vi "9604 String to Integer Overflow--error.vi"(7 "Type":T1(ring), 8 "error in":errorcluster, 11 "Integer String":string) -> (0 "error out":errorcluster)   [LabVIEW 2020, in "CANopen.lvlib"]
uses:
  CANopen.lvlib
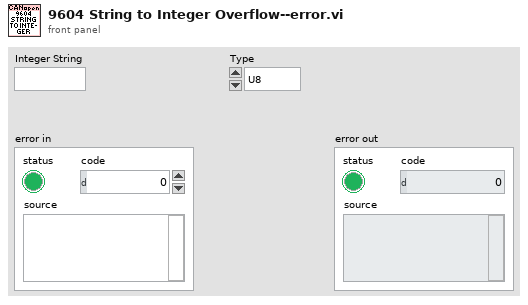
[diagram p1: front panel]
types:
  T1 = enum16{"U8", "U16", "U32", "I8", "I16", "I32", "I64", "U64"}
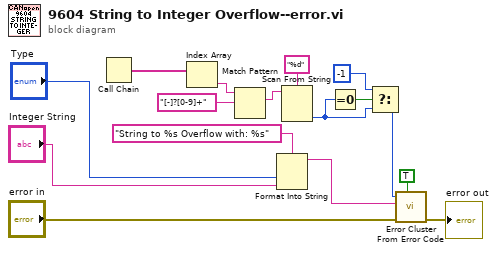
[diagram p0: block diagram]
diagram:
  n1 = Call Chain() -> (call chain=w9:string[])
  n2 = Index Array(array=w9) -> (element=w3:string)  [unwired: 1 in]
  n3 = Match Pattern(string=w3, regular expression="[-]?[0-9]+") -> (match substring=w2:string)  [unwired: 1 in, 3 out]
  n4 = Format Into String(format string="String to %s Overflow with: %s" ("error message (\"\")"), "Type", "Integer String") -> (resulting string=w13:string)  [unwired: 2 in, 1 out]
  n5 = Scan From String(format string="%d", input string=w2) -> (output 1=w6:i32)  [unwired: 3 in, 3 out]
  n6 = Equal To 0?(x=w6) -> (x = 0?=w5:bool)
  n7 = Select(t=-1, s=w5, f=w6) -> (s? t:f=w8:i32)
  n8 = call <vilib>:"Error Cluster From Error Code.vi"("show call chain? (False)"=TRUE, "error in (no error)"="error in", "error message (\"\")"=w13, "error code (0)"=w8) -> ("error out"=→"error out":errorcluster)  [unwired: 5 in]
